vi "Dashboard Main.vi"() -> ()   [LabVIEW 2015]
uses:
  Common Code/Auton Command Cluster.ctl
  Common Code/Auton File Lists.ctl
  Vision/Camera Types.ctl
  Common Code/Goal Vision Packet.ctl
  <vilib>/Rock Robotics/WPI/Camera/WPI_CameraSettings Read MJPG.ctl
  <vilib>/Rock Robotics/WPI/Camera/WPI_CameraImageSize.ctl
  Common Code/Encoder Values Super Cluster.ctl
  Common Code/Encoder Values.ctl
  Common Code/Power and Diagnostic Data.ctl
  Common Code/Utilities/PDP Data.ctl
  Common Code/Utilities/PCM Data.ctl
  Common Code/IMU Data.ctl
  navX.Library.v2/navX Library v2/TypeDefs/Flags/Z900_navX_Flags_CalibrationStatusTypeDef.ctl
  navX.Library.v2/navX Library v2/TypeDefs/Flags/Z900_navX_Flags_OpStatusTypeDef.ctl
  Common Code/Intake Status Cluster.ctl
  Common Code/Intake Mode.ctl
  Common Code/Intake States.ctl
  Common Code/Climb Status Cluster.ctl
  Common Code/Climb Mode.ctl
  Common Code/Climb Presets.ctl
  Common Code/Major Loop Times.ctl
  Common Code/Shooter State Cluster.ctl
  Common Code/Shooter State.ctl
  Common Code/Shoot Modes Enum.ctl
  Common Code/Shot Type.ctl
  Common Code/Drivetrain Settings.ctl
  Common Code/Shooter Presets.ctl
  Common Code/Shot Presets.ctl
  Common Code/Intake Presets.ctl
  Common Code/Drivetrain Output Range.ctl
  Common Code/Ultrasonic Data.ctl
  Common Code/Autonomous Presets.ctl
  Common Code/Robot Name.ctl
  Common Code/Encoder Control.ctl
  Common Code/Drivetrain Status Cluster.ctl
  Common Code/Drivetrain Modes.ctl
  Common Code/Dist Drive Status.ctl
  Common Code/Auto Shift Cluster.ctl
  Common Code/Dashboard Communication/Dashboard Control Data.ctl
  Common Code/Dashboard Drivetrain Command.ctl
  Common Code/Drivetrain Vision.ctl
  Common Code/Ball Tracking Command Cluster.ctl
  Common Code/Ball Vision Packet.ctl
  Common Code/Tracking Mode.ctl
  Common Code/IntakeEcoderControl.ctl
  Common Code/Enabled Systems.ctl
  Common Code/Dashboard Communication/Dashboard Display Data.ctl
  <vilib>/Rock Robotics/WPI/Dashboard/WPI_DashboardLogging Global.vi
  <vilib>/Utility/inputDevices.llb/keyboardAcquire.vi
  navX.Library.v2/navX Library v2/navX Library v2.lvlib
panel:
  in  "Robot":T1
  in  "Logging Filename":path=path ""
  in  "stop":bool
  out "DumbDashMessage":string="137 values loaded OK"
  in  "Save":bool
  in  "Load":bool
  in  "TCP":refnum<k5>
  in  "Rec Mode":enum32{"Stop", "Record", "Playback"}(radio)
  out "Image Message":string="Timeout in Camera Communications"
  in  "Dashboard Tab":T2(tab)
  out "Auto Shift Enabled?":bool
  out "Gear":dbl
  out "Pressure":dbl
  out "Goal Active? 2":bool
  out "Drivetrain Mode":bool
  out "Intake State":bool
  out "Right RPM":dbl(knob) scale=0.0..5000.0
  out "Left RPM":dbl(knob) scale=0.0..5000.0
  out "Mode":T3(ring)=enum."Disconnected"
  out "Shooter Mode":bool
  out "Gyro":dbl(knob) scale=0.0..360.0 scale format="%#.7g"
  out "Climb Mode":bool
  out "Intake Mode":bool
  out "Shooter State":bool
  out "Camera IP":string="0.0.0.0"
  out "Robot IP":string="0.0.0.0"
  out "Angle Ready?":bool
  out "RPM Ready?":bool
  out "Vision Ready?":bool
  out "Ball Loaded?":bool
  out "Shooter Ready?":bool
  out "Front Camera Display":T4(plugin-control)
  in  "Camera Mode":u16(ring)=3 items=["Camera Off", "USB Camera SW", "USB Camera HW", "IP Camera"]
  out "FPS":dbl
  out "Bandwidth (Mbps)":dbl
  out "navX Calibration Status":T5 items=["IMU_CAL_STATE_MASK"=3, "IMU_CAL_STATE_INPROGRESS"=0, "IMU_CAL_STATE_ACCUMULATE"=1, "IMU_CAL_STATE_COMPLETE"=2]
  out "Front Camera Display 2":T4(plugin-control)
  out "Line Number":i32
  in  "Auton Presets":T6
  out "Auton Command Cluster":T7
  out "Auton File Lists":T8
  in  "Auto-Shift":T9
  in  "Encoder Settings":T10
  in  "Drivetrain Settings":T11={"Gyro Tolerance"=6.0, "Throttle Ramp (ms)"=250.0, "Kv"=0.0, "Ka"=0.0, "Feed Forward P"=1.0, "Feed Forward D"=0.0, "Goal Vision PID gains"={"proportional gain (Kc)"=0.8, "integral time (Ti, min)"=0.05, "derivative time (Td, min)"=0.003}, "Goal Detection Window"=12.0, "Creep Rate"=0.0, "Vision Throttle Threshold"=0.0, "Min Turn Output"=0.0, "Left Batter Angle"=0.0, "Right Batter Angle"=0.0} {"Goal Vision PID gains"."derivative time (Td, min)" format="%.5f"; "Goal Vision PID gains"."integral time (Ti, min)" format="%.3f"; "Goal Vision PID gains"."proportional gain (Kc)" format="%.3f"}
  in  "Goal Output Range":cluster{"output high":dbl, "output low":dbl}={"output high"=0.8, "output low"=-0.8}
  out "Encoder Values":T12
  in  "Steer PID output":cluster{"output high":dbl, "output low":dbl}
  in  "Steer PID gains":T14
  out "Drivetrain Status Cluster":T15={"Modes"=enum."Manual", "Y (Throttle)"=0.0, "X (Steer)"=0.0, "Gyro In Range?"=FALSE, "Distance Drive Finished?"=FALSE, "Stop Eject Lockout"=FALSE, "Dist Drive Status"={"Y In Range"=FALSE, "X In Range"=FALSE, "Gyro In Range"=FALSE, "Y Dist"=0.0, "X Dist"=0.0, "Gyro"=0.0}, "Y Target"=0.0, "Heading Target"=0.0, "Vision Target Aligned?"=FALSE, "Gear"=0.0, "1st Gear Time"=0.0, "2nd Gear Time"=0.0, "1st Gear Shifts"=0.0, "2nd Gear Shifts"=0.0} {"2nd Gear Time" scale=0.0..135.0; "1st Gear Time" scale=0.0..135.0}
  in  "Shooter Presets":T18={"Batter Shot"={"L"=1450.0, "R"=1450.0, "A"=69.0}, "Deep Middle"={"L"=0.0, "R"=0.0, "A"=0.0}, "Manual Shot"={"L"=1000.0, "R"=1000.0, "A"=0.0}, "Left Ticks Per Rotation"=-409.6, "Right Ticks Per Rotation"=409.6, "Low Bar Shot"={"L"=2100.0, "R"=2100.0, "A"=42.0}, "Shooter RPM Tolerance"=100.0, "Trigger Power"=0.9, "Fire from Load Delay"=250, "Max Angle"=80.0, "Min Angle"=42.0, "Angle PID gains"={"P"=1.0, "I"=0.0, "D"=0.002}, "Angle Output"={"output high"=0.5, "output low"=-0.5}, "Shooter Angle Tolerance"=3.0, "Vision Shoot x^2"=0.0, "Vision Shoot x"=0.0, "Feed Forward Max Accel"=160.57, "Feed Forward Kv"=0.000217, "Backwards Trigger"=-0.6, "Shot Finish Delay (ms)"=250.0, "Angle Max Current"=40.0, "Angle Current Trip Time"=500.0, "Intake Angle"=80.0, "Vision Shoot c"=0.0, "Reset?"=FALSE, "Button Release Delay"=0.0, "Angle Pot x"=7.0746, "Angle Pot c"=33.439, "Ignore Angle?"=FALSE, "Max RPM"=4600.0, "Safty Frist Angle"=44.0, "Intake Danger Height"=35.0, "Angle Pot B"=0, "Angle Pot M"=12.0, "FF Finish RPM"=0.0, "RPM PID Right"={"P"=0.17, "I"=0.0, "D"=0.0, "FF"=0.036}, "RPM PID Left"={"P"=0.18, "I"=0.0, "D"=0.0, "FF"=0.037}, "Backwards RPM"=-300.0, "Vision RPM"=0.0, "Run Wheels Backward Delay"=0, "Cleat Shot"={"L"=0.0, "R"=0.0, "A"=0.0}, "Vision Far RPM"=0.0, "Vision Far Distance"=0.0, "Vision Far Angle"=0.0}
  out "Shooter State Cluster":T20 {"Trigger Output" scale=-1.0..1.0; "Angle Motor Output" scale=-1.0..1.0; "Right RPM" scale=0.0..5000.0; "Left RPM" scale=0.0..5000.0}
  in  "Intake Presets":T24={"Intake Speed"=0.8, "Outake Speed"=-0.8, "Low Height"=5.0, "Half Height"=55.0, "High Idle Height"=90.0, "Angle Speed"=0.0, "Angle Tolerance"=5.0, "Encoder Scale"=0.001478, "Load Height"=4.0, "Output Range"={"output high"=0.4, "output low"=-0.4}, "Rotation Power Max/Min"=0.5, "MaxCurrent"=40.0, "Intake Trip Time"=500.0, "Idle Height"=27.0, "Max Height"=90.0, "Reset Encoders?"=FALSE, "PID gains"={"proportional gain (Kc)"=1.0, "integral time (Ti, min)"=0.0, "derivative time (Td, min)"=0.003}, "Intake Stop Delay"=0, "Settle Time"=0.0, "Settle Wait Time"=0.0, "Pull Up Delay"=0.0} {"Pull Up Delay" format="%#_7g"; "Settle Wait Time" format="%#_7g"; "Settle Time" format="%#_7g"; "Intake Stop Delay" format="%#_7g"; "Max Height" format="%#_7g"; "Idle Height" format="%#_7g"; "Intake Trip Time" format="%#_7g"; "MaxCurrent" format="%#_7g"; "Rotation Power Max/Min" format="%#_7g"; "Load Height" format="%#_7g"; "Encoder Scale" format="%#_7g"; "Angle Tolerance" format="%#_7g"; "Angle Speed" format="%#_7g"; "High Idle Height" format="%#_7g"; "Half Height" format="%#_7g"; "Low Height" format="%#_7g"; "Outake Speed" format="%#_7g"; "Intake Speed" format="%#_7g"}
  out "Intake Status Cluster":T26
  in  "Climb Presets":T29={"Pull Power"=0.0, "Extend Power"=1.0}
  out "Climb Status Cluster":T30
  in  "Pressure B":dbl
  in  "Pressure M":dbl=22.0
  out "Pressure Sensor Voltage":dbl
  out "IMU Data":T32 {"OP Status" items=["INITIALIZING", "SELFTEST_IN_PROGRESS", "ERROR", "IMU_AUTOCAL_IN_PROGRESS", "NORMAL"]; "Calibration Status" items=["IMU_CAL_STATE_MASK"=3, "IMU_CAL_STATE_INPROGRESS"=0, "IMU_CAL_STATE_ACCUMULATE"=1, "IMU_CAL_STATE_COMPLETE"=2]}
  out "Gyro 2":dbl(knob) scale=0.0..360.0 scale format="%#.7g"
  out "Ultrasonic Data":T34
  out "Ball Cam Active?":bool
  out "Camera Display 2":T4(plugin-control)
  in  "Aspect Fudge Factor":dbl=1.0
  in  "Score Threshold 2":dbl=75.0 format="%#_13g"
  out "Goal Display":T4(plugin-control)
  out "Found Targets":T35(array[cluster]) {"Normalized Rect"."Numeric 5" format="%#_2g"; "Normalized Rect"."Numeric 3" format="%#_2g"; "Normalized Rect"."Numeric 2" format="%#_2g"; "Normalized Rect"."Numeric" format="%#_2g"}
  in  "Camera Type":T36=enum."1013"
  out "Goal Vision Packet":T37
  in  "Goal Camera Settings":T38={"fps"=30, "compression"=30, "Image Size"=enum."320x240"}
  in  "File number":i32
  in  "Use Goal File?":bool
  in  "Color Components":T40={"Hue"={34.0, 185.0}, "Sat"={0.0, 181.0}, "Val"={142.0, 255.0}} {"Val" scale=0.0..255.0; "Sat" scale=0.0..255.0; "Hue" scale=0.0..255.0 scale format="%#_3g"}
  out "Goal Active?":bool
  in  "Camera Mode 2":u16(ring) items=["Camera Off", "USB Camera SW", "USB Camera HW", "IP Camera"]
  out "FPS 2":dbl
  out "Bandwidth (Mbps) 2":dbl
  in  "Ball Camera Settings":T38={"fps"=30, "compression"=30, "Image Size"=enum."320x240"}
  out "Front Camera Display 3":T4(plugin-control)
  in  "Vision Timeout":dbl
  out "Power and Diagnostic Data":T41
  out "Control Info":T44
  out "Status Info":T45
  out "DS TCP":T46={"Error Strings"="", "Disable Counts"={0, 0}, "Rail Faults"={0, 0, 0}, "Robot IP"="0.0.0.0", "DB Mode"=4, "Event Info"={"Name"="", "Type"=0, "Number"=0, "Replay"=0}, "Camera Addr"="0.0.0.0"}
  out "Robot Metrics":T47
  out "Loop Times":T48
  # "USB Cam"
  # "Axis Cam"
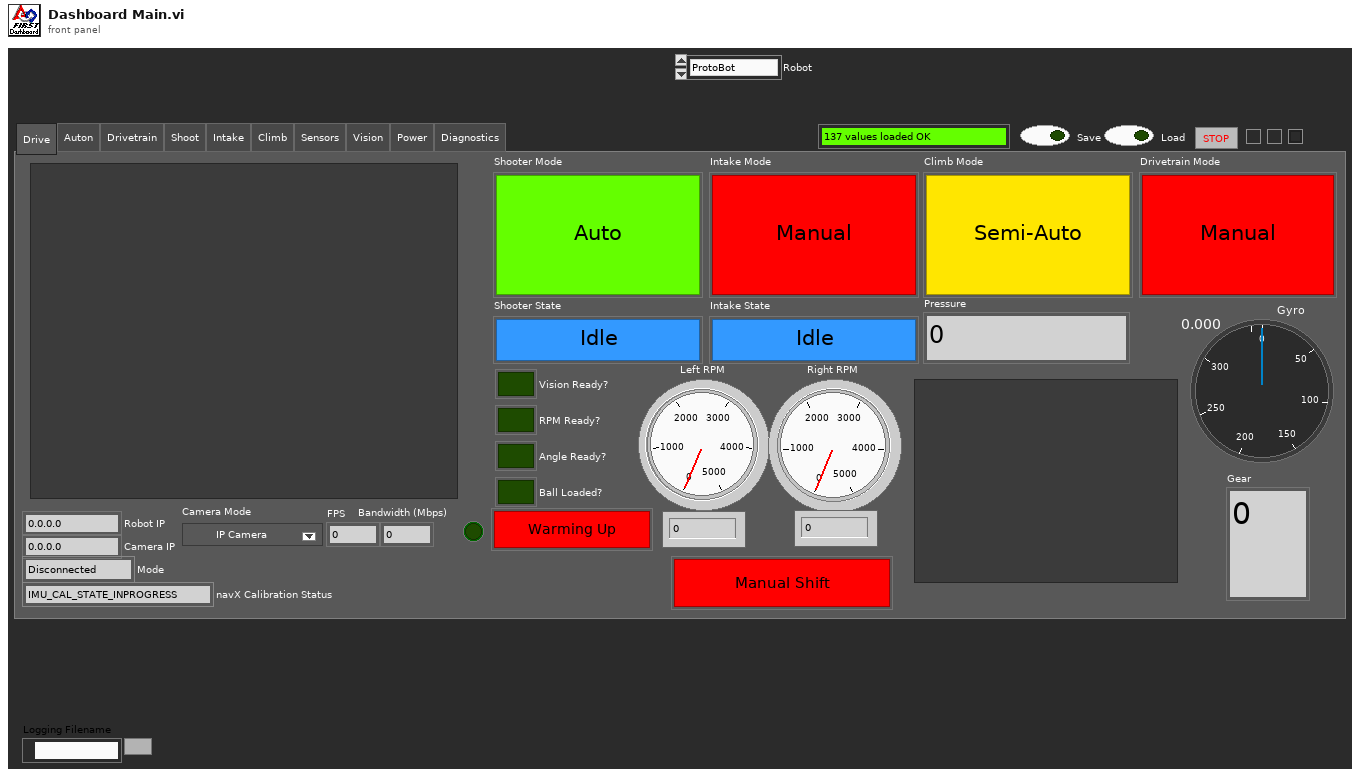
[diagram p1: front panel]
types:
  T1 = typedef "Robot Name.ctl" = enum16{"ProtoBot", "Main Robot", "Practice Robot"}
  T2 = enum32{"Drive", "Auton", "Drivetrain", "Shoot", "Intake", "Climb", "Sensors", "Vision", "Power", "Diagnostics"}
  T3 = enum8{"Tele-Op Disabled", "Tele-Op Enabled", "Auto Disabled", "Auto Enabled", "Test Disabled", "Test Enabled", "Disconnected", "No Code", "E-Stop"}
  T4 = typedef "IMAQ Image.ctl" = refnum<image>
  T5 = typedef "navX Library v2.lvlib/Z900_navX_Flags_CalibrationStatusTypeDef.ctl" = u8
  T6 = typedef "Autonomous Presets.ctl" = cluster{"Pitch Limit":dbl, "Roll Limit":dbl, "Start Position":dbl, "Cross Position":dbl}
  T7 = typedef "Auton Command Cluster.ctl" = cluster{"Command ID":i32, "maxTime":dbl, "Y Distance":dbl, "Heading":dbl, "Throttle":dbl, "Async":dbl, "Velocity":dbl, "Acceleration":dbl, "To":dbl, "Condition":dbl, "Shot Type":dbl, "Left RPM":dbl, "Override RPM":i32, "Override Angle":i32, "Right RPM":dbl, "Angle":dbl, "Intake Mode":i32, "Intake Cmd":i32, "Intake O":i32, "Eject O":i32, "Angle O":i32, "Arm O":i32, "Intake Speed":dbl, "Eject Speed":dbl, "Arm Angle":dbl, "Arm Speed":dbl, "Intake?":i32, "Eject?":i32, "Left":dbl, "Right":dbl, "Pivot Speed":dbl, "Y Dist":dbl, "Position":dbl, "Desired Position":i32, "Shooter Mode":dbl, "Shooter Command":dbl}
  T8 = typedef "Auton File Lists.ctl" = cluster{"Current Queue":string, "General Scripts":string, "Defense Scripts":string, "Movement Scripts":string}
  T9 = typedef "Auto Shift Cluster.ctl" = cluster{"Delay":dbl, "Speed Thresh":dbl, "Upshift Accel":dbl, "Upshift Throttle":dbl, "Upshift Throttle Accel":dbl, "Downshift Throttle":dbl, "Downshift Throttle Accel":dbl}
  T10 = typedef "Encoder Control.ctl" = cluster{"Right Tick Constant":dbl, "Left Tick Constant":dbl, "Reset?":bool, "Y Dist":cluster{"PID gains":cluster{"proportional gain (Kc)":dbl, "integral time (Ti, min)":dbl, "derivative time (Td, min)":dbl}}, "Y Stop Thresh":dbl, "Y Stop Speed":dbl}
  T11 = typedef "Drivetrain Settings.ctl" = cluster{"Gyro Tolerance":dbl, "Throttle Ramp (ms)":dbl, "Kv":dbl, "Ka":dbl, "Feed Forward P":dbl, "Feed Forward D":dbl, "Goal Vision PID gains":cluster{"proportional gain (Kc)":dbl, "integral time (Ti, min)":dbl, "derivative time (Td, min)":dbl}, "Goal Detection Window":dbl, "Creep Rate":dbl, "Vision Throttle Threshold":dbl, "Min Turn Output":dbl, "Left Batter Angle":dbl, "Right Batter Angle":dbl}
  T12 = typedef "Encoder Values Super Cluster.ctl" = cluster{"Left Encoder":T13, "Right Encoder":T13}
  T13 = typedef "Encoder Values.ctl" = cluster{"Distance":dbl, "Speed":dbl, "Ticks":dbl}
  T14 = cluster{"proportional gain (Kc)":dbl, "integral time (Ti, min)":dbl, "derivative time (Td, min)":dbl}
  T15 = typedef "Drivetrain Status Cluster.ctl" = cluster{"Modes":T16, "Y (Throttle)":dbl, "X (Steer)":dbl, "Gyro In Range?":bool, "Distance Drive Finished?":bool, "Stop Eject Lockout":bool, "Dist Drive Status":T17, "Y Target":dbl, "Heading Target":dbl, "Vision Target Aligned?":bool, "Gear":dbl, "1st Gear Time":dbl, "2nd Gear Time":dbl, "1st Gear Shifts":dbl, "2nd Gear Shifts":dbl}
  T16 = typedef "Drivetrain Modes.ctl" = enum16{"Tank", "Climb", "Manual", "Goal Vision Targeting", "PID Distance Drive", "Hybrid", "Gyro Steer"}
  T17 = typedef "Dist Drive Status.ctl" = cluster{"Y In Range":bool, "X In Range":bool, "Gyro In Range":bool, "Y Dist":dbl, "X Dist":dbl, "Gyro":dbl}
  T18 = typedef "Shooter Presets.ctl" = cluster{"Batter Shot":T19, "Deep Middle":T19, "Manual Shot":T19, "Left Ticks Per Rotation":dbl, "Right Ticks Per Rotation":dbl, "Low Bar Shot":T19, "Shooter RPM Tolerance":dbl, "Trigger Power":dbl, "Fire from Load Delay":i32, "Max Angle":dbl, "Min Angle":dbl, "Angle PID gains":cluster{"P":dbl, "I":dbl, "D":dbl}, "Angle Output":cluster{"output high":dbl, "output low":dbl}, "Shooter Angle Tolerance":dbl, "Vision Shoot x^2":dbl, "Vision Shoot x":dbl, "Feed Forward Max Accel":dbl, "Feed Forward Kv":dbl, "Backwards Trigger":dbl, "Shot Finish Delay (ms)":dbl, "Angle Max Current":dbl, "Angle Current Trip Time":dbl, "Intake Angle":dbl, "Vision Shoot c":dbl, "Reset?":bool, "Button Release Delay":dbl, "Angle Pot x":dbl, "Angle Pot c":dbl, "Ignore Angle?":bool, "Max RPM":dbl, "Safty Frist Angle":dbl, "Intake Danger Height":dbl, "Angle Pot B":i32, "Angle Pot M":dbl, "FF Finish RPM":dbl, "RPM PID Right":cluster{"P":dbl, "I":dbl, "D":dbl, "FF":dbl}, "RPM PID Left":cluster{"P":dbl, "I":dbl, "D":dbl, "FF":dbl}, "Backwards RPM":dbl, "Vision RPM":dbl, "Run Wheels Backward Delay":u32, "Cleat Shot":T19, "Vision Far RPM":dbl, "Vision Far Distance":dbl, "Vision Far Angle":dbl}
  T19 = typedef "Shot Presets.ctl" = cluster{"L":dbl, "R":dbl, "A":dbl}
  T20 = typedef "Shooter State Cluster.ctl" = cluster{"State":T21, "Left RPM":dbl, "Right RPM":dbl, "Shooter Ready?":bool, "Ball Loaded?":bool, "Current Angle":dbl, "Angle Motor Output":dbl, "Trigger Output":dbl, "Angle Ready?":bool, "RPM Ready?":bool, "Vision Ready?":bool, "Ball Loaded?":bool, "Mode":T22, "Shot Type":T23, "Pot Height":dbl, "Current Tripped Forward?":bool, "Current Tripped Backward?":bool, "Right Servo":i32, "Left Servo":i32, "IR Override":bool, "Intake Danger?":bool, "Intake Angle Ready?":bool}
  T21 = typedef "Shooter State.ctl" = enum16{"Idle", "Settle Ball", "Warmup", "Shooter Ready", "Shoot"}
  T22 = typedef "Shoot Modes Enum.ctl" = enum16{"Manual", "Safe", "Auto"}
  T23 = typedef "Shot Type.ctl" = enum16{"Batter Shot", "Corner Shot", "Cleat Shot", "Vision Shot", "Deep Middle Shot"}
  T24 = typedef "Intake Presets.ctl" = cluster{"Intake Speed":dbl, "Outake Speed":dbl, "Low Height":dbl, "Half Height":dbl, "High Idle Height":dbl, "Angle Speed":dbl, "Angle Tolerance":dbl, "Encoder Scale":dbl, "Load Height":dbl, "Output Range":T25, "Rotation Power Max/Min":dbl, "MaxCurrent":dbl, "Intake Trip Time":dbl, "Idle Height":dbl, "Max Height":dbl, "Reset Encoders?":bool, "PID gains":cluster{"proportional gain (Kc)":dbl, "integral time (Ti, min)":dbl, "derivative time (Td, min)":dbl}, "Intake Stop Delay":u32, "Settle Time":dbl, "Settle Wait Time":dbl, "Pull Up Delay":dbl}
  T25 = typedef "Drivetrain Output Range.ctl" = cluster{"output high":dbl, "output low":dbl}
  T26 = typedef "Intake Status Cluster.ctl" = cluster{"Roller Power":dbl, "Angle Power":dbl, "Intake Mode":T27, "Intake States":T28, "Rollers Active?":bool, "Current Height":dbl, "Target Height":dbl, "Encoder Raw Position":dbl, "Forward Tripped?":bool, "Backward Tripped?":bool, "Override IR?":bool}
  T27 = typedef "Intake Mode.ctl" = enum16{"Safe", "Auto", "Manual"}
  T28 = typedef "Intake States.ctl" = enum16{"Idle", "Set roller speed", "Move to angle", "Go Hard or Go Home", "Ball Settle"}
  T29 = typedef "Climb Presets.ctl" = cluster{"Pull Power":dbl, "Extend Power":dbl}
  T30 = typedef "Climb Status Cluster.ctl" = cluster{"Pull Power":dbl, "Unpin Power":dbl, "PTO Engaged?":bool, "Climb Mode":T31}
  T31 = typedef "Climb Mode.ctl" = enum16{"Auto", "Semi-Auto", "Manual"}
  T32 = typedef "IMU Data.ctl" = cluster{"Pitch":sgl, "Roll":sgl, "Yaw":sgl, "Data Valid?":bool, "Temp":sgl, "MOVING":bool, "YAW_STABLE":bool, "Accel X":sgl, "Accel Y":sgl, "Accel Z":sgl, "Accel Magnitude":sgl, "Pitch Rate":sgl, "Roll Rate":sgl, "Yaw Rate":sgl, "NavX Opened?":bool, "Calibration Status":T5, "OP Status":T33}
  T33 = typedef "navX Library v2.lvlib/Z900_navX_Flags_OpStatusTypeDef.ctl" = u8
  T34 = typedef "Ultrasonic Data.ctl" = cluster{"Left Ultrasonic":dbl, "Right Ultrasonic":dbl}
  T35 = cluster{"Distance (ft)":dbl, "Center":cluster{dbl, dbl}, "Normalized Rect":cluster{"Numeric":dbl, "Numeric 2":dbl, "Numeric 3":dbl, "Numeric 5":dbl}}[]
  T36 = typedef "Camera Types.ctl" = enum16{"206", "1011", "1013", "MS HD3000 square", "MS HD3000 640x480"}
  T37 = typedef "Goal Vision Packet.ctl" = cluster{"Distance":dbl, "Center X":dbl, "Center Y":dbl, "Found Target?":bool, "Robot Center":dbl, "Angle":dbl}
  T38 = typedef "WPI_CameraSettings Read MJPG.ctl" = cluster{"fps":i32, "compression":i32, "Image Size":T39}
  T39 = typedef "WPI_CameraImageSize.ctl" = enum16{"640x480", "320x240", "160x120", "Custom"}
  T40 = cluster{"Hue":cluster{dbl, dbl}, "Sat":cluster{dbl, dbl}, "Val":cluster{dbl, dbl}}
  T41 = typedef "Power and Diagnostic Data.ctl" = cluster{"PDP Data":T42, "PCM Data":T43, "roboRIO input voltage (V)":dbl, "roboRIO input current (A)":dbl, "3.3V Rail Short":bool, "5 V Rail Short":bool, "6 V Rail Short":bool, "roboRIO Brownout":bool, "Outputs Enabled?":bool}
  T42 = typedef "PDP Data.ctl" = cluster{"Battery Voltage":sgl, "Temperature (degrees C)":sgl, "Internal Battery R (Ohms)":sgl, "Energy (J)":sgl, "Power (W)":sgl, "Total Current (A)":sgl, "Battery Voltage Fault":bool, "Temperature Fault":bool, "Hardware Fault":bool, "Currents":cluster{"[0]":sgl, "[1]":sgl, "[2]":sgl, "[3]":sgl, "[4]":sgl, "[5]":sgl, "[6]":sgl, "[7]":sgl, "[8]":sgl, "[9]":sgl, "[10]":sgl, "[11]":sgl, "[12]":sgl, "[13]":sgl, "[14]":sgl, "[15]":sgl}, "Current Faults":cluster{"[0]":bool, "[1]":bool, "[2]":bool, "[3]":bool, "[4]":bool, "[5]":bool, "[6]":bool, "[7]":bool, "[8]":bool, "[9]":bool, "[10]":bool, "[11]":bool, "[12]":bool, "[13]":bool, "[14]":bool, "[15]":bool}}
  T43 = typedef "PCM Data.ctl" = cluster{"Compressor Fault":bool, "Solenoid Fault":bool, "Compressor Enabled":bool, "Hardware Fault":bool, "Compressor Current":dbl}
  T44 = cluster{"Control Bits":cluster{"TestMode":bool, "Autonomous":bool, "Enabled":bool, "FMS Present":bool, bool, bool, bool, "E-Stop":bool}, "Team Station ":u8, "Countdown":sgl, "Joystick Values":cluster{"Axes":dbl[], "Buttons":bool[], "POVs":i16[]}[]}
  T45 = cluster{"Status bits":cluster{"Test Mode":bool, "Autonomous":bool, "Enabled":bool, "Code Start":bool, "Brownout":bool, "Reserved 2":bool, "Reserved 3":bool, "E-Stop":bool}, "Code Trace":cluster{"Disabled":bool, "TeleOp":bool, "Auto":bool, "Test":bool}, "Controller Type":enum16{"unknown", "cRIO", "roboRio"}, "Code?":enum16{"unknown", "noCode", "code"}, "Battery V":dbl}
  T46 = cluster{"Error Strings":string, "Disable Counts":cluster{u16, u16}, "Rail Faults":cluster{u16, u16, u16}, "Robot IP":string, "DB Mode":u8, "Event Info":cluster{"Name":string, "Type":u8, "Number":u16, "Replay":u8}, "Camera Addr":string}
  T47 = cluster{"Storage":cluster{"Disk Free":u64, "RAM Block":u32, "RAM free":u32}, "CPU Utilization":cluster{"CPU % ISR":sgl, "CPU % Time Crit":sgl, "CPU % Timed Str":sgl, "CPU % High":sgl, "CPU % Above":sgl, "CPU % Normal":sgl, "CPU % Low":sgl}, "CAN":cluster{"% Bus Utilization":sgl, "Bus Off Cnt":u32, "TX_FIFO Full Cnt":u32, "Receive Error Cnt":u8, "Transmit Error Cnt":u8}, "HID":cluster{"HID Outputs":u32, "Rumble Low":u16, "Rumble High":u16}[]}
  T48 = typedef "Major Loop Times.ctl" = cluster{"DT Loop Timer":u32, "Shooter Loop Timer":u32, "Intake Loop Timer":u32, "US Loop Timer":u32, "Auton File Loop Timer":u32}
  T49 = typedef "Image Type" = u32
  T50 = typedef "NI_LVConfig.lvlib/Config Data RefNum.ctl" = refnum<k1>
  T51 = cluster{cluster{dbl, dbl}, cluster{dbl, dbl}, cluster{dbl, dbl}}
  T52 = cluster{"Bounding box":cluster{"left":dbl, "top":dbl, "right":dbl, "bottom":dbl}, "Aspect Ratio":dbl, "Area to CH":dbl, "X Mask":dbl, "Y Mask":dbl, "Moment":dbl}[]
  T53 = cluster{"Distance (ft)":dbl, "Center":cluster{dbl, dbl}, "Normalized Rect":cluster{"Numeric":dbl, "Numeric 2":dbl, "Numeric 3":dbl, "Numeric 5":dbl}}
  T54 = typedef "Dashboard Display Data.ctl" = cluster{"Auton Command Cluster":T7, "Auton File Lists":T8, "Drivetrain Status Cluster":T15, "Encoder Values":T12, "IMU Data":T32, "Power and Diagnostic Data":T41, "Gyro":dbl, "Shooter State Cluster":T20, "Intake Status Cluster":T26, "Ultrasonic Data":T34, "Climb Status Cluster":T30, "Loop Times":T48, "Pressure":dbl, "Pressure Voltage":dbl, "Auton Line Number":i32, "Autoshift Enabled":bool}
  T55 = typedef "Dashboard Control Data.ctl" = cluster{"Shooter Presets":T18, "Encoder Control":T10, "Steer PID output":cluster{"output high":dbl, "output low":dbl}, " Steer PID gains":cluster{"proportional gain (Kc)":dbl, "integral time (Ti, min)":dbl, "derivative time (Td, min)":dbl}, "Drivetrain Settings":T11, "Vision Packet":T37, "Dashboard Drivetrain Command":T56, "Info/Command Cluster":T58, "Ball Vision Packet":T59, "Intake Presets":T24, "Intake Encoder Control":T61, "Climb Presets":T29, "Goal Output Range":cluster{"output high":dbl, "output low":dbl}, "Enabled Systems":T62, "Auton Presets":T6, "Pressure M":dbl, "Pressure B":dbl, "Vision Timeout":dbl, "Auto-Shift":T9}
  T56 = typedef "Dashboard Drivetrain Command.ctl" = cluster{"Drivetrain Vision":T57}
  T57 = typedef "Drivetrain Vision.ctl" = cluster{"Goal Window":dbl, "Ball Window":dbl}
  T58 = typedef "Ball Tracking Command Cluster.ctl" = cluster{"Distance to Ball":dbl, "Desired Angle":dbl, "Command":enum16{"Turn to Ball", "Turn to Angle", "Get Distance"}, "Pixels from Center":dbl}
  T59 = typedef "Ball Vision Packet.ctl" = cluster{"Ball Detected?":bool, "Distance to Ball":dbl, "Desired Angle":dbl, "Pixels from Center":dbl, "Tracking mode":T60}
  T60 = typedef "Tracking Mode.ctl" = enum16{"Turn to Ball", "Turn to Angle"}
  T61 = typedef "IntakeEcoderControl.ctl" = cluster{"Arm Tick Constant":dbl, "Reset?":bool, "Y Dist":cluster{"PID gains":cluster{"proportional gain (Kc)":dbl, "integral time (Ti, min)":dbl, "derivative time (Td, min)":dbl}}, "Y Stop Thresh":dbl, "Y Stop Speed":dbl}
  T62 = typedef "Enabled Systems.ctl" = cluster{"Shoot":bool, "Intake":bool, "DT":bool, "Gyro":bool, "100ms":bool, "US":bool}
  T63 = cluster{"Image Size":bool, "Image Type":bool, "Pixel Value":bool, "ROI Information":bool, "Zoom Factor":bool}
  T64 = enum16{"0", "1", "2", "3", "4", "5", "6", "7", "8", "9", "A", "B", "C", "D", "E", "F", "G", "H", "I", "J", "K", "L", "M", "N", "O", "P", "Q", "R", "S", "T", "U", "V", "W", "X", "Y", "Z", "F1", "F2", "F3", "F4", "F5", "F6", "F7", "F8", "F9", "F10", "F11", "F12", "F13", "F14", "F15", "ADD", "BACK", "BACKSLASH", "CAPITAL", "COMMA", "DECIMAL", "DELETE", "DIVIDE", "DOWN", "END", "EQUALS", "ESCAPE", "GRAVE (`)", "HOME", "INSERT", "LBRACKET", "LCONTROL", "LEFT", "L ALT", "LSHIFT", "LWIN", "MINUS", "MULTIPLY", "NEXT", "NUMLOCK", "NUMPAD_0", "NUMPAD_1", "NUMPAD_2", "NUMPAD_3", "NUMPAD_4", "NUMPAD_5", "NUMPAD_6", "NUMPAD_7", "NUMPAD_8", "NUMPAD_9", "PAUSE", "PERIOD", "PRIOR (PG UP)", "RBRACKET", "RCONTROL", "RETURN", "RIGHT", "R ALT", "RSHIFT", "RWIN", "SCROLL", "SEMICOLON", "SLASH", "SPACE", "SUBTRACT", "TAB", "UP", "ENTER (num pad)", "' (quote)"}[]
  T65 = typedef "DumbDash Control.ctl" = cluster{"Name":string, "Ref":refnum<vi>, "Type":T66}
  T66 = typedef "DumbDash Control Type.ctl" = enum16{"Invalid", "Number", "Boolean", "String"}
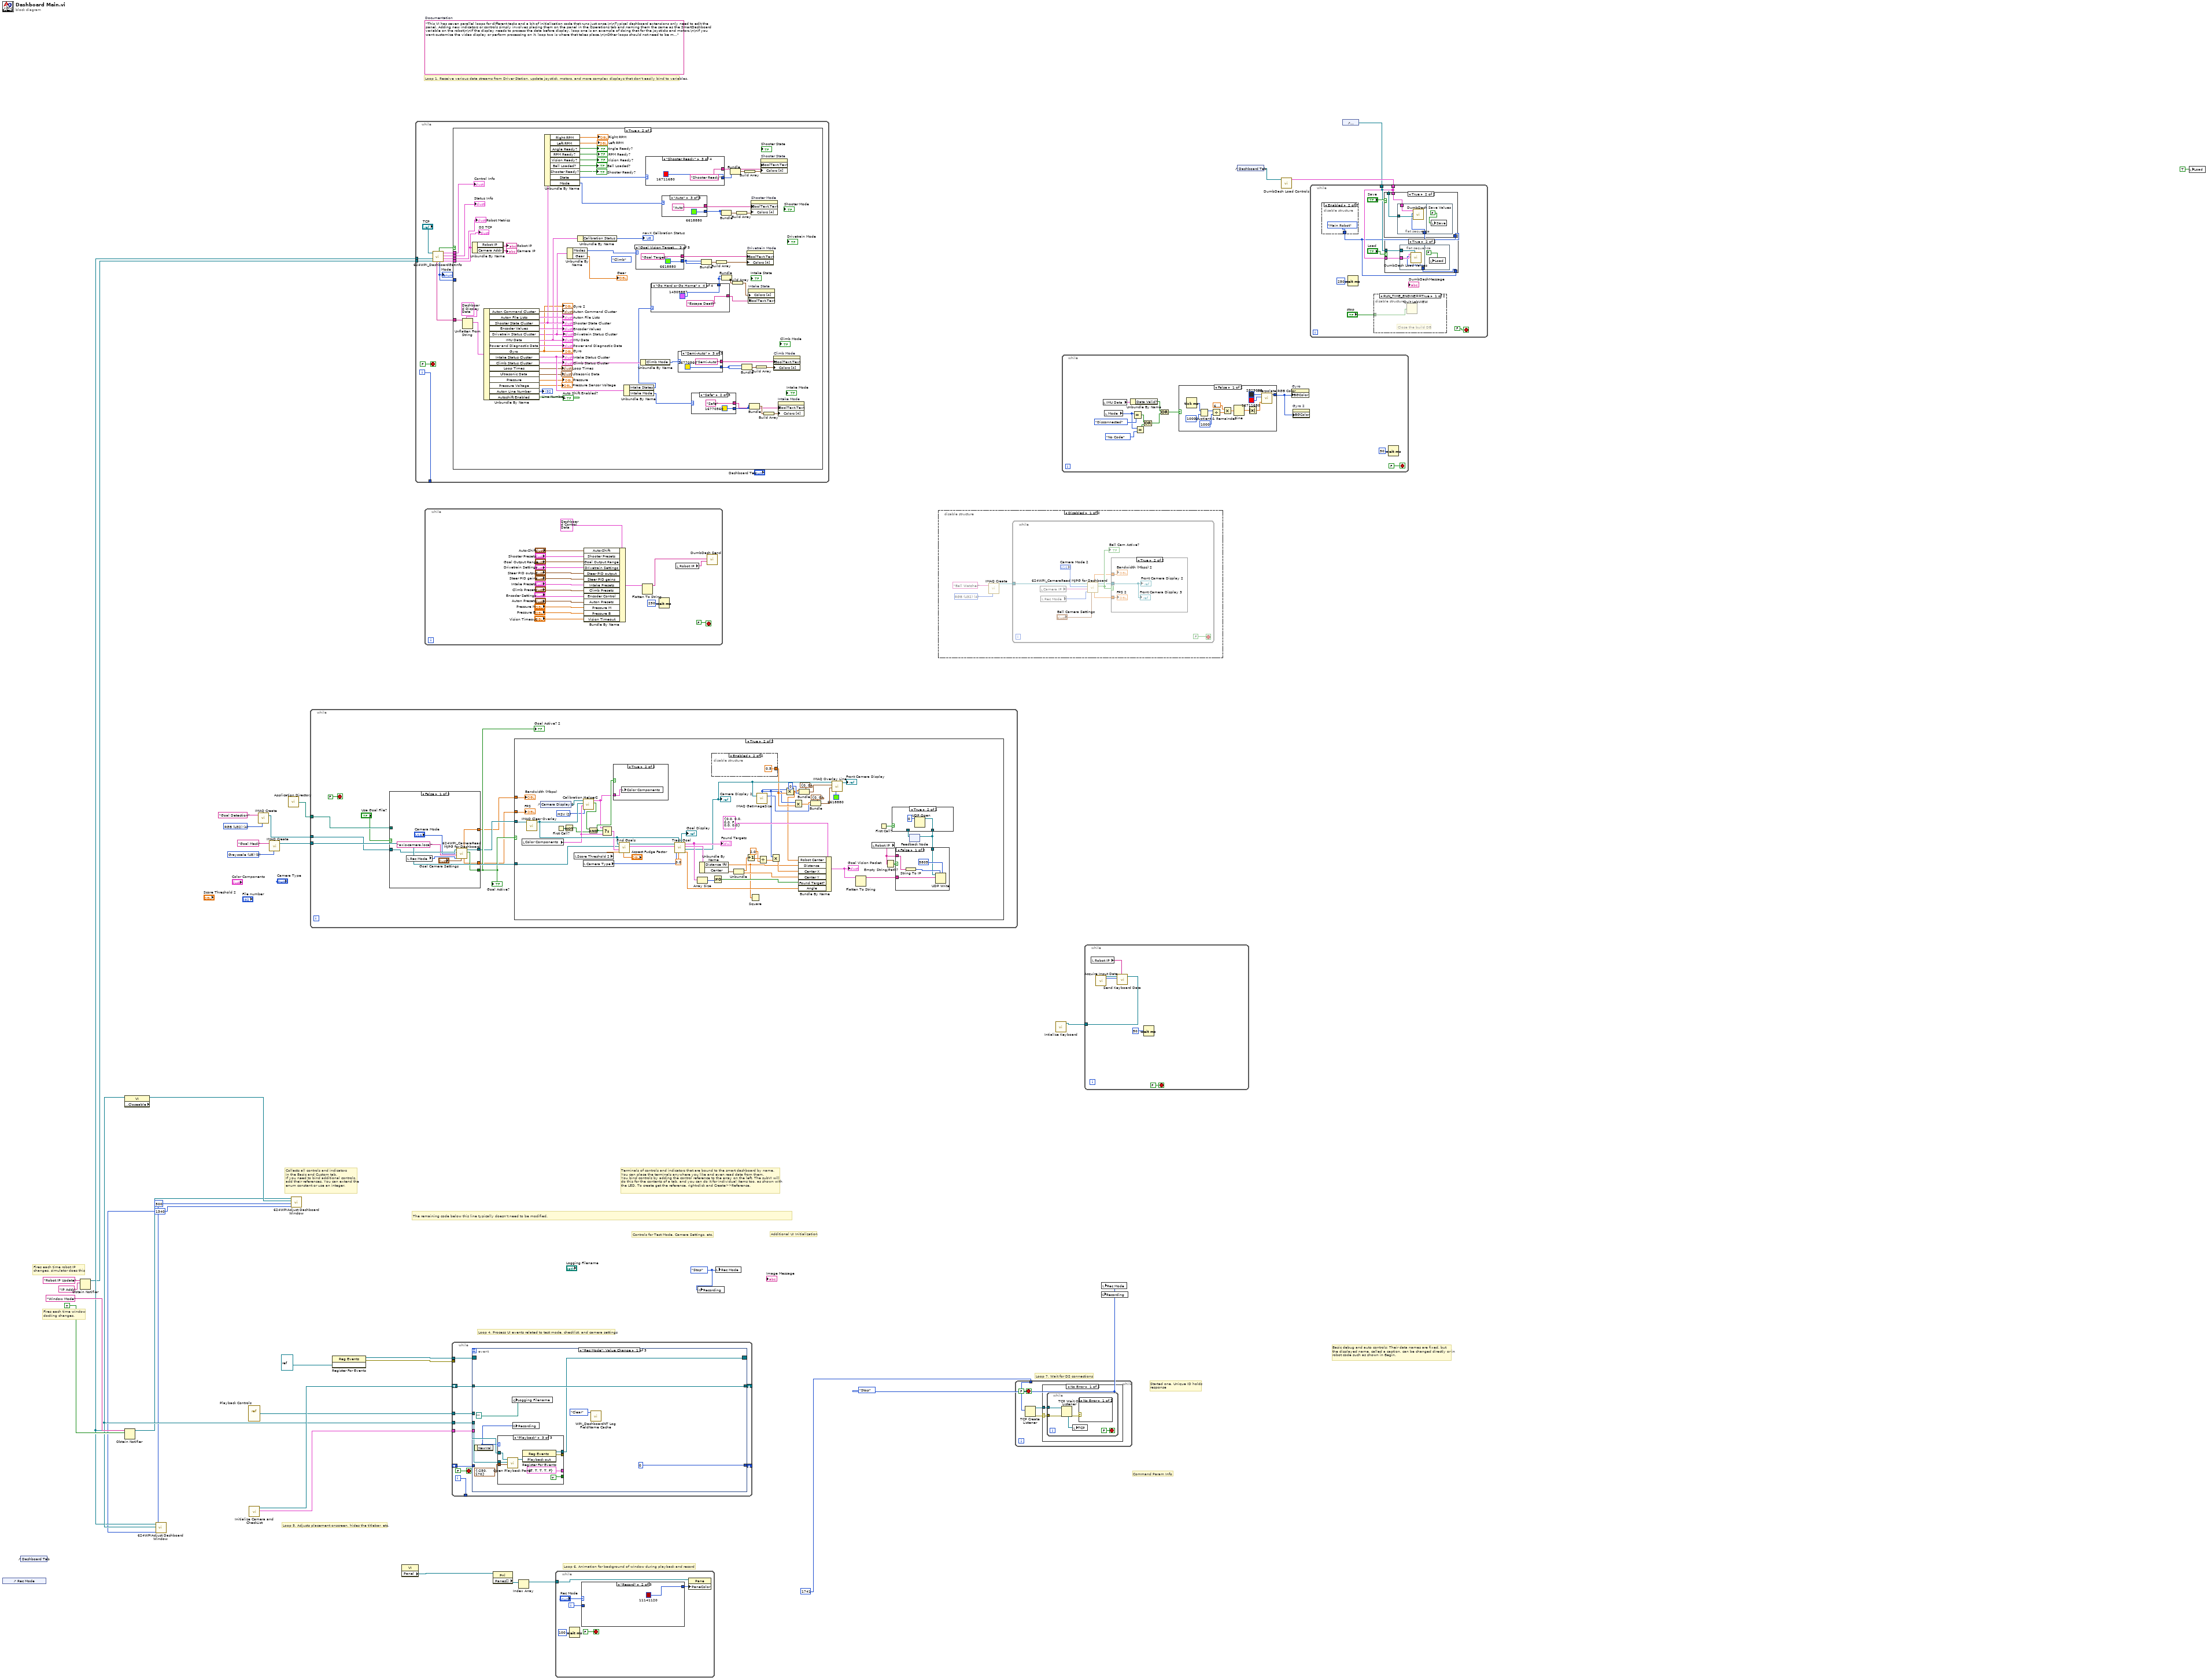
[diagram p0: block diagram]
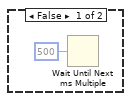
[diagram p2: hidden frame]
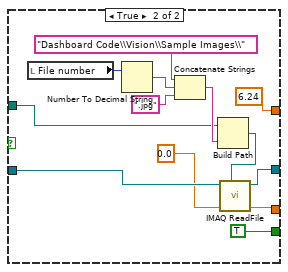
[diagram p4: hidden frame]
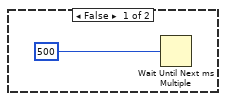
[diagram p5: hidden frame]
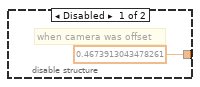
[diagram p9: hidden frame]
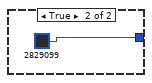
[diagram p10: hidden frame]
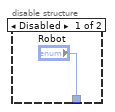
[diagram p11: hidden frame]
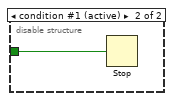
[diagram p12: hidden frame]
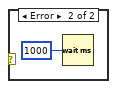
[diagram p15: hidden frame]
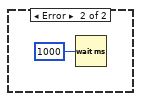
[diagram p16: hidden frame]
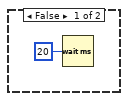
[diagram p17: hidden frame]
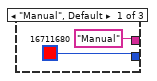
[diagram p18: hidden frame]
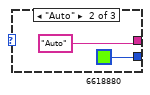
[diagram p19: hidden frame]
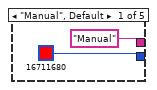
[diagram p20: hidden frame]
diagram:
  w3 = T49 0 items=["Grayscale (U8)", "Grayscale (I16)", "Grayscale (SGL)", "Complex (CSG)", "RGB (U32)", "HSL (U32)", "RGB (U64)", "Grayscale (U16)"] ("Image Type")
  w7 = T49 4 items=["Grayscale (U8)", "Grayscale (I16)", "Grayscale (SGL)", "Complex (CSG)", "RGB (U32)", "HSL (U32)", "RGB (U64)", "Grayscale (U16)"] ("Image Type")
  w10 = enum16{"Stop", "Record", "Playback"}."Stop"
  w15 = 1340
  w16 = 500
  w20 = enum32{"Stop", "Record", "Playback"}."Stop" ("Rec Mode")
  (unwired) "This VI has seven parallel loops for different tasks and a bit of initialization code that runs just once.\n\nTypical dashboard extensions only need to edit the panel. Adding new indicators or controls simply involves placing them on the panel in the Operations tab and naming them the same as the SmartDashboard variable on the robot\n\nIf the display needs to process the data before display, loop one is an example of doing that for the joysticks and motors.\n\nIf you want customize the video display or perform processing on it, loop two is where that takes place.\n\nOther loops should not need to be modified. They are pretty standard, and document the task they perform."  # Documentation
  # "Command Param Info"
  # "Started one, Unique ID holds\nresponse"
  # "Loop 7. Wait for DS connections"
  # "Basic debug and auto controls: Their data names are fixed, but\nthe displayed name, called a caption, can be changed directly or in\nrobot code such as shown in Begin."
  # "Controls for Test Mode, Camera Settings, etc."
  # "Additional UI Initialization"
  # "Loop 6. Animation for background of window during playback and record"
  # "Fires each time robot IP\nchanges, simulator does this"
  # "Fires each time window\ndocking changes."
  # "Collects all controls and indicators\nin the Basic and Custom tab.\nIf you need to bind additional controls,\nadd their references. You can extend the\nenum constant or use an integer."
  # "The remaining code below this line typically doesn't need to be modified."
  # "Loop 4. Process UI events related to test mode, checklist, and camera settings"
  # "Terminals of controls and indicators that are bound to the smart dashboard by name.\nYou can place the terminals anywhere you like and even read data from them.\nYou bind controls by adding the control reference to the array on the left. The subVI will\ndo this for the contents of a tab, and you can do it for individual items too, as shown with\nthe LED. To create get the reference, right-click and Create>>Reference."
  # "Loop 5. Adjusts placement onscreen, hides the titlebar, etc."
  # "Loop 1. Receive various data streams from Driver Station, update joystick, motors, and more complex displays that don't easily bind to variables."
  n1 = control-ref of="Rec Mode"() -> ()  [unwired: 1 out]
  n2 = control-ref of="Dashboard Tab"() -> ()  [unwired: 1 out]
  n3 = Obtain Notifier(name (unnamed)="Robot IP Update", notification data type="IP Addr" ("name (unnamed)")) -> (notifier out=w14:refnum<notifier>)  [unwired: 2 in, 2 out]
  n4 = property class="VI" props=["Front Panel.Closeable"]() -> (reference out=w19:refnum<vi>)  [unwired: 2 in, 2 out]
  n5 = Obtain Notifier(name (unnamed)="Window Mode", notification data type=TRUE) -> (notifier out=w18:refnum<notifier>)  [unwired: 2 in, 2 out]
  n6 = call "624WPIAdjust Dashboard Window.vi"("Width"=w15, "Height"=w16, "VI"=w19, "Notifier in"=w18) -> ()  [unwired: 8 in]
  n7 = vi-ref "Playback Controls.vi"() -> (w24:refnum<vi>)
  n8 = call "Initialize Camera and CheckList.vi"() -> ("Array"=w29:cluster{string[]}[], "File Refnum"=w28:T50)  [unwired: 9 in, 1 out]
  n9 = call "IMAQ Create"("Image Name"="Goal Detection", "Image Type"=w7) -> ("New Image"=w8:T4)  [unwired: 3 in, 1 out]
  n10 = call "IMAQ Create"("Image Name"="Goal Mask", "Image Type"=w3) -> ("New Image"=w5:T4)  [unwired: 3 in, 1 out]
  n11 = call <vilib>:"Application Directory.vi"() -> ("Application Directory"=w2:path)
  n12 = call "624WPIAdjust Dashboard Window.vi"("Width"=w15, "Height"=w16, "VI"=w19, "Notifier in"=w18) -> ()  [unwired: 8 in]
  n13 = while {
    tunnel: w5 -> [w42]
    tunnel: w8 -> [w40]
    tunnel: w2 -> [w38]
    stop <- FALSE stop-if-true
    n14 = case shown="False" "Use Goal File?" {
      tunnel: [w46 TRUE] -> w41
      tunnel: w40 -> [w51 w62]
      tunnel: [w45 w61] -> w39
      tunnel: w38 -> [_ w56]
      tunnel: [w43 6.24 ("Bandwidth (Mbps)")] -> w36
      tunnel: [w44 0.0 ("FPS")] -> w35
      frame False {
        n15 = local read "Rec Mode"() -> (w48:enum32{"Stop", "Record", "Playback"})
        n16 = call "624WPI_CameraRead MJPG for Dashboard.vi"("Camera Settings"="Goal Camera Settings", "Rec Mode"=w48, "Camera IP"="axis-camera.local", "Camera Mode"="Camera Mode", "Refnum in"=w51) -> ("Active"=w46:bool, "Refnum out"=w45:T4, "FPS"=w44:dbl, "Bandwidth (Mbps)"=w43:dbl)  [unwired: 3 in]
      }
      frame True {
        n17 = local read "File number"() -> (w54:i32)
        n18 = Number To Decimal String(number=w54) -> (decimal integer string=w59:string)  [unwired: 1 in]
        n19 = Concatenate Strings("Dashboard Code\\Vision\\Sample Images\\", w59, ".jpg" ("string")) -> (w57:string)
        n20 = Build Path(base path=w56, name or relative path=w57) -> (appended path=w55:path)
        n21 = call "IMAQ ReadFile"("File Path"=w55, "Image"=w62) -> ("Image Out"=w61:T4)  [unwired: 5 in, 4 out]
      }
    }
    "Goal Active?" <- w41
    "Goal Active? 2" <- w41
    n22 = case shown="True" w41 {
      tunnel: w39 -> [_ w118]
      tunnel: w42 -> [_ w99]
      tunnel: w36 -> [_ w107]
      tunnel: w35 -> [_ w106]
      frame False {
        n23 = Wait Until Next ms Multiple(millisecond multiple=u32 500) -> ()  [unwired: 1 out]
      }
      frame True {
        w102 = u16 2 items=["RGB", "HSL", "HSV", "HSI", "CIE L*a*b*", "CIE XYZ"] ("Color Mode")
        n24 = local read "Color Components"() -> (w103:T40)
        n25 = call "IMAQ Clear Overlay"("Image"=w118) -> ("Image Out"=w105:T4)  [unwired: 9 in, 1 out]
        n26 = control-ref of="Camera Display 2"() -> (w104:refnum<vi>)
        n27 = First Call?() -> (First Call?: T/F=w69:bool)
        n28 = Not(x=w69) -> (.not. x?=w68:bool)
        n29 = local read "Score Threshold 2"() -> (w119:dbl)
        n30 = call "Calibration Helper2.vi"("Color Mode"=w102, "Color Components"=w103, "Image"=w105, "Image Ctl Refnum"=w104) -> ("Changed"=w67:bool, "output color"=w65:T51)  [unwired: 6 in]
        n31 = local read "Camera Type"() -> (w115:T36)
        n32 = And(x=w67, y=w68) -> (x .and. y?=w66:bool)
        n33 = Select(t=w65, s=w66, f=w103) -> (s? t:f=w101:T40)
        n34 = case shown="True" w66 {
          tunnel: w65 -> [_ w120]
          frame False {
          }
          frame True {
            n35 = local write "Color Components"(w120) -> ()
          }
        }
        n36 = call "Find Goals.vi"("Aspect Fudge Factor"="Aspect Fudge Factor", "Score Threshold"=w119, "Color"=w101, "Image Dst"=w99, "Image Src"=w105) -> ("Targets"=w117:T52, "Masked Image"=w116:T4)  [unwired: 5 in]
        n37 = call "Track Goal.vi"("Offset"=0.0, "Original Image"=w105, "Camera Type"=w115, "Targets"=w117, "Goal Display"=w116) -> ("Angle Difference"=w81:dbl, "Target Line Masking Out"=w90:T4, "Best Target Available"=w114:T53, "Found Targets"=w109:T35, "Goal Display"=→"Goal Display":T4)  [unwired: 2 in]
        "Found Targets" <- w109
        "Camera Display 2" <- w90
        n38 = Array Size(array=w109) -> (size(s)=w110:i32)
        n39 = Unbundle By Name(w114) -> ("Distance (ft)"=w78:dbl, "Center"=w112:cluster{dbl, dbl})
        n40 = disable-structure shown="Enabled" {
          disable-tunnel: [0.4673913043478261 0.5] -> w89
          frame Disabled {
            # "when camera was offset"
          }
          frame Enabled {
          }
        }
        n41 = Not Equal To 0?(x=w110) -> (x != 0?=w108:bool)
        n42 = Unbundle(w112) -> (w88:dbl, w111:dbl)
        n43 = Increment(x=w88) -> (x+1=w87:dbl)
        n44 = Square(x=w78) -> ()  [unwired: 1 out]
        n45 = call "IMAQ GetImageSize"("Image"=w90) -> ("Y Resolution"=w92:i32, "X Resolution"=w83:i32)  [unwired: 3 in, 1 out]
        n46 = Divide(x=w87, y=2.0) -> (x/y=w85:dbl)
        n47 = Multiply(x=w83, y=w85) -> (x*y=w84:dbl)
        n48 = Multiply(x=w83, y=w89) -> (x*y=w82:dbl)
        n49 = Multiply(x=w83, y=w89) -> (x*y=w95:dbl)
        n50 = Bundle By Name(cluster=T37 {"Distance"=0.0, "Center X"=0.0, "Center Y"=0.0, "Found Target?"=FALSE, "Robot Center"=0.0, "Angle"=0.0}, "Robot Center"=w82, "Distance"=w78, "Center X"=w84, "Center Y"=w111, "Found Target?"=w108, "Angle"=w81) -> (w71:T37)
        "Goal Vision Packet" <- w71
        n51 = Bundle(cluster=cluster{"X":i32, "Y":i32} {"X"=0, "Y"=0} ("Start Point"), "X"=w82, "Y"=0) -> (w94:cluster{"X":i32, "Y":i32})
        n52 = Bundle(cluster=cluster{"X":i32, "Y":i32} {"X"=0, "Y"=0} ("Start Point"), "X"=w95, "Y"=w92) -> (w93:cluster{"X":i32, "Y":i32})
        n53 = call "IMAQ Overlay Line"("Color"=u32 6618880, "End Point"=w93, "Start Point"=w94, "Image"=w90) -> ("Image Out"=→"Front Camera Display":T4)  [unwired: 6 in, 1 out]
        n54 = Flatten To String(anything=w71) -> (data string=w70:string)  [unwired: 3 in, 2 out]
        n55 = local read "Robot IP"() -> (w72:string)
        n56 = First Call?() -> (First Call?: T/F=w75:bool)
        n57 = Empty String/Path?(string/path=w72) -> (empty?=w76:bool)
        n58 = feedback #1() -> (w73:refnum<k16>)  [unwired: 1 in]
        n59 = case shown="True" w75 {
          tunnel: [w121 w123] -> w74
          tunnel: w73 -> [w121 _]
          frame False {
          }
          frame True {
            n60 = UDP Open(11:u16 0 ("port")) -> (port=w123:refnum<k16>)  [unwired: 4 in, 2 out]
          }
        }
        n61 = case shown="False" w76 {
          tunnel: w72 -> [w126 _]
          tunnel: w70 -> [w125 _]
          tunnel: w74 -> [w124 _]
          frame False {
            n62 = String To IP(1:w126) -> (0:w127:u32)
            n63 = UDP Write(address=w127, port or service name=u16 5805, connection ID=w124, data in=w125) -> ()  [unwired: 2 in, 2 out]
          }
          frame True {
            # "The robot IP is not\nready yet, don't try\nto send data"
          }
        }
        n64 = feedback-in #1(w74) -> ()
        "Bandwidth (Mbps)" <- w107
        "FPS" <- w106
      }
    }
  }
  n65 = register-events(refnum<vi> refnum) -> (reference out=w23:refnum<event-registration>, error out=w22:errorcluster)  [unwired: 2 in]
  n66 = property class="VI"() -> ("Panel"=w26:refnum<vi>)  [unwired: 2 in, 2 out]
  n67 = while {
    tunnel: [w141] -> _
    tunnel: w14 -> [w140]
    tunnel: w18 -> [w138]
    i -> [w141]
    stop <- FALSE stop-if-true
    n68 = call "624WPI_DashboardGetInfo.vi"("Binding Refnum"=w140, "Window Mode Notifier"=w138, "TCP Cnx"="TCP") -> ("Power and Errors"=w137:T46, "Robot Metrics"=w136:T47, "Status Info"=w135:T45, "Control Info"=w134:T44, "Robot Mode"=w133:T3, "Process?"=w132:bool, "Custom Dashboard Data"=w131:string)  [unwired: 2 in]
    "Mode" <- w133
    n69 = case shown="True" w132 {
      tunnel: w135 -> [_ w206]
      tunnel: w136 -> [_ w205]
      tunnel: w134 -> [_ w207]
      tunnel: w137 -> [_ w204]
      tunnel: w133 -> [_ _]
      tunnel: w131 -> [_ w201]
      frame False {
        n70 = Wait (ms)(milliseconds to wait=u32 20) -> ()  [unwired: 1 out]
      }
      frame True {
        (unwired) Drivetrain_Modes."Climb" ("Modes")
        n71 = Unflatten From String(type=T54 {"Auton Command Cluster"={"Command ID"=0, "maxTime"=0.0, "Y Distance"=0.0, "Heading"=0.0, "Throttle"=0.0, "Async"=0.0, "Velocity"=0.0, "Acceleration"=0.0, "To"=0.0, "Condition"=0.0, "Shot Type"=0.0, "Left RPM"=0.0, "Override RPM"=0, "Override Angle"=0, "Right RPM"=0.0, "Angle"=0.0, "Intake Mode"=0, "Intake Cmd"=0, "Intake O"=0, "Eject O"=0, "Angle O"=0, "Arm O"=0, "Intake Speed"=0.0, "Eject Speed"=0.0, "Arm Angle"=0.0, "Arm Speed"=0.0, "Intake?"=0, "Eject?"=0, "Left"=0.0, "Right"=0.0, "Pivot Speed"=0.0, "Y Dist"=0.0, "Position"=0.0, "Desired Position"=0, "Shooter Mode"=0.0, "Shooter Command"=0.0}, "Auton File Lists"={"Current Queue"="", "General Scripts"="", "Defense Scripts"="", "Movement Scripts"=""}, "Drivetrain Status Cluster"={"Modes"=enum."Manual", "Y (Throttle)"=0.0, "X (Steer)"=0.0, "Gyro In Range?"=FALSE, "Distance Drive Finished?"=FALSE, "Stop Eject Lockout"=FALSE, "Dist Drive Status"={"Y In Range"=FALSE, "X In Range"=FALSE, "Gyro In Range"=FALSE, "Y Dist"=0.0, "X Dist"=0.0, "Gyro"=0.0}, "Y Target"=0.0, "Heading Target"=0.0, "Vision Target Aligned?"=FALSE, "Gear"=0.0, "1st Gear Time"=0.0, "2nd Gear Time"=0.0, "1st Gear Shifts"=0.0, "2nd Gear Shifts"=0.0}, "Encoder Values"={"Left Encoder"={"Distance"=0.0, "Speed"=0.0, "Ticks"=0.0}, "Right Encoder"={"Distance"=0.0, "Speed"=0.0, "Ticks"=0.0}}, "IMU Data"={"Pitch"=0.0, "Roll"=0.0, "Yaw"=0.0, "Data Valid?"=FALSE, "Temp"=0.0, "MOVING"=FALSE, "YAW_STABLE"=FALSE, "Accel X"=0.0, "Accel Y"=0.0, "Accel Z"=0.0, "Accel Magnitude"=0.0, "Pitch Rate"=0.0, "Roll Rate"=0.0, "Yaw Rate"=0.0, "NavX Opened?"=FALSE, "Calibration Status"=0, "OP Status"=0}, "Power and Diagnostic Data"={"PDP Data"={"Battery Voltage"=0.0, "Temperature (degrees C)"=0.0, "Internal Battery R (Ohms)"=0.0, "Energy (J)"=0.0, "Power (W)"=0.0, "Total Current (A)"=0.0, "Battery Voltage Fault"=FALSE, "Temperature Fault"=FALSE, "Hardware Fault"=FALSE, "Currents"={"[0]"=0.0, "[1]"=0.0, "[2]"=0.0, "[3]"=0.0, "[4]"=0.0, "[5]"=0.0, "[6]"=0.0, "[7]"=0.0, "[8]"=0.0, "[9]"=0.0, "[10]"=0.0, "[11]"=0.0, "[12]"=0.0, "[13]"=0.0, "[14]"=0.0, "[15]"=0.0}, "Current Faults"={"[0]"=FALSE, "[1]"=FALSE, "[2]"=FALSE, "[3]"=FALSE, "[4]"=FALSE, "[5]"=FALSE, "[6]"=FALSE, "[7]"=FALSE, "[8]"=FALSE, "[9]"=FALSE, "[10]"=FALSE, "[11]"=FALSE, "[12]"=FALSE, "[13]"=FALSE, "[14]"=FALSE, "[15]"=FALSE}}, "PCM Data"={"Compressor Fault"=FALSE, "Solenoid Fault"=FALSE, "Compressor Enabled"=FALSE, "Hardware Fault"=FALSE, "Compressor Current"=0.0}, "roboRIO input voltage (V)"=0.0, "roboRIO input current (A)"=0.0, "3.3V Rail Short"=FALSE, "5 V Rail Short"=FALSE, "6 V Rail Short"=FALSE, "roboRIO Brownout"=FALSE, "Outputs Enabled?"=FALSE}, "Gyro"=0.0, "Shooter State Cluster"={"State"=enum."Idle", "Left RPM"=0.0, "Right RPM"=0.0, "Shooter Ready?"=FALSE, "Ball Loaded?"=FALSE, "Current Angle"=0.0, "Angle Motor Output"=0.0, "Trigger Output"=0.0, "Angle Ready?"=FALSE, "RPM Ready?"=FALSE, "Vision Ready?"=FALSE, "Ball Loaded?"=FALSE, "Mode"=enum."Manual", "Shot Type"=enum."Batter Shot", "Pot Height"=0.0, "Current Tripped Forward?"=FALSE, "Current Tripped Backward?"=FALSE, "Right Servo"=0, "Left Servo"=0, "IR Override"=FALSE, "Intake Danger?"=FALSE, "Intake Angle Ready?"=FALSE}, "Intake Status Cluster"={"Roller Power"=0.0, "Angle Power"=0.0, "Intake Mode"=enum."Auto", "Intake States"=enum."Idle", "Rollers Active?"=FALSE, "Current Height"=0.0, "Target Height"=0.0, "Encoder Raw Position"=0.0, "Forward Tripped?"=FALSE, "Backward Tripped?"=FALSE, "Override IR?"=FALSE}, "Ultrasonic Data"={"Left Ultrasonic"=0.0, "Right Ultrasonic"=0.0}, "Climb Status Cluster"={"Pull Power"=0.0, "Unpin Power"=0.0, "PTO Engaged?"=FALSE, "Climb Mode"=enum."Auto"}, "Loop Times"={"DT Loop Timer"=0, "Shooter Loop Timer"=0, "Intake Loop Timer"=0, "US Loop Timer"=0, "Auton File Loop Timer"=0}, "Pressure"=0.0, "Pressure Voltage"=0.0, "Auton Line Number"=0, "Autoshift Enabled"=FALSE}, binary string=w201) -> (value=w186:T54)  [unwired: 3 in, 2 out]
        n72 = Unbundle By Name(w204) -> ("Robot IP"=→"Robot IP":string, "Camera Addr"=→"Camera IP":string)
        n73 = Unbundle By Name(w186) -> ("Auton Command Cluster"=→"Auton Command Cluster":T7, "Auton File Lists"=→"Auton File Lists":T8, "Shooter State Cluster"=w177:T20, "Encoder Values"=→"Encoder Values":T12, "Drivetrain Status Cluster"=w146:T15, "IMU Data"=w171:T32, "Power and Diagnostic Data"=→"Power and Diagnostic Data":T41, "Gyro"=→"Gyro" →"Gyro 2":dbl, "Intake Status Cluster"=w185:T26, "Climb Status Cluster"=w179:T30, "Loop Times"=→"Loop Times":T48, "Ultrasonic Data"=→"Ultrasonic Data":T34, "Pressure"=→"Pressure":dbl, "Pressure Voltage"=→"Pressure Sensor Voltage":dbl, "Auton Line Number"=→"Line Number":i32, "Autoshift Enabled"=→"Auto Shift Enabled?":bool)
        "IMU Data" <- w171
        "Intake Status Cluster" <- w185
        "Climb Status Cluster" <- w179
        "Shooter State Cluster" <- w177
        "Drivetrain Status Cluster" <- w146
        n74 = Unbundle By Name(w177) -> ("Right RPM"=→"Right RPM":dbl, "Left RPM"=→"Left RPM":dbl, "Angle Ready?"=→"Angle Ready?":bool, "RPM Ready?"=→"RPM Ready?":bool, "Vision Ready?"=→"Vision Ready?":bool, "Ball Loaded?"=→"Ball Loaded?":bool, "Shooter Ready?"=→"Shooter Ready?":bool, "State"=w196:T21, "Mode"=w195:T22)
        n75 = Unbundle By Name(w146) -> ("Modes"=w162:T16, "Gear"=→"Gear":dbl)
        n76 = Unbundle By Name(w171) -> ("Calibration Status"=→"navX Calibration Status":T5)
        n77 = Unbundle By Name(w185) -> ("Intake States"=w166:T28, "Intake Mode"=w182:T27)
        n78 = case shown="\"Goal Vision Targeting\"" w162 {
          tunnel: ["Manual" "Climb" "Goal Target" "PID Drive" "Hybrid Drive"] -> w160
          tunnel: [u32 16711680 u32 16770560 u32 6618880 u32 9263615 u32 16743698] -> w161
          frame "Manual", Default {
          }
          frame "Climb" {
          }
          frame "Goal Vision Targeting" {
          }
          frame "PID Distance Drive" {
          }
          frame "Hybrid" {
          }
        }
        n79 = Unbundle By Name(w179) -> ("Climb Mode"=w153:T31)
        n80 = case shown="\"Shooter Ready\"" w196 {
          tunnel: ["Idle" "Warmup" "Shooter Ready" "Shooting"] -> w191
          tunnel: [u32 3381759 u32 16746240 u32 16711680 u32 6618880] -> w194
          frame "Idle", Default {
          }
          frame "Warmup" {
          }
          frame "Shooter Ready" {
          }
          frame "Shoot" {
          }
        }
        n81 = case shown="\"Go Hard or Go Home\"" w166 {
          tunnel: ["Idle" "Rolling Rollers" "Moving to Angle" "Escape Death"] -> w170
          tunnel: [u32 3381759 u32 16746240 u32 16711680 u32 14309887] -> w169
          frame "Idle", Default {
          }
          frame "Set roller speed" {
          }
          frame "Move to angle" {
          }
          frame "Go Hard or Go Home" {
          }
        }
        n82 = case shown="\"Auto\"" w195 {
          tunnel: ["Manual" "Safe" "Auto"] -> w199
          tunnel: [u32 16711680 u32 16770560 u32 6618880] -> w200
          frame "Manual", Default {
          }
          frame "Safe" {
          }
          frame "Auto" {
          }
        }
        n83 = case shown="\"Semi-Auto\"" w153 {
          tunnel: ["Manual" "Auto" "Semi-Auto"] -> w157
          tunnel: [u32 16711680 u32 6618880 u32 16770560] -> w154
          frame "Manual", Default {
          }
          frame "Auto" {
          }
          frame "Semi-Auto" {
          }
        }
        n84 = case shown="\"Safe\"" w182 {
          tunnel: ["Manual" "Safe" "Auto"] -> w180
          tunnel: [u32 16711680 u32 16770560 u32 6618880] -> w183
          frame "Manual", Default {
          }
          frame "Safe" {
          }
          frame "Auto" {
          }
        }
        n85 = Bundle(w161, w161) -> (w158:cluster{u32, u32})  [unwired: 1 in]
        n86 = Build Array(w158) -> (w159:cluster{u32, u32}[])
        n87 = Bundle(w200, w200) -> (w197:cluster{u32, u32})  [unwired: 1 in]
        n88 = Bundle(w169, w169) -> (w168:cluster{u32, u32})  [unwired: 1 in]
        n89 = Bundle(w194, w194) -> (w193:cluster{u32, u32})  [unwired: 1 in]
        n90 = Build Array(w168) -> (w167:cluster{u32, u32}[])
        n91 = Build Array(w197) -> (w198:cluster{u32, u32}[])
        n92 = Bundle(w154, w154) -> (w155:cluster{u32, u32})  [unwired: 1 in]
        n93 = Build Array(w193) -> (w192:cluster{u32, u32}[])
        n94 = property on="Drivetrain Mode" class="Bool (strict)"("BoolText.Text"=w160, "Colors [4]"=w159) -> ()  [unwired: 2 in, 2 out]
        n95 = property on="Intake State" class="Bool (strict)"("Colors [4]"=w167, "BoolText.Text"=w170) -> ()  [unwired: 2 in, 2 out]
        n96 = Bundle(w183, w183) -> (w184:cluster{u32, u32})  [unwired: 1 in]
        n97 = property on="Shooter Mode" class="Bool (strict)"("BoolText.Text"=w199, "Colors [4]"=w198) -> ()  [unwired: 2 in, 2 out]
        n98 = Build Array(w155) -> (w156:cluster{u32, u32}[])
        n99 = property on="Shooter State" class="Bool (strict)"("BoolText.Text"=w191, "Colors [4]"=w192) -> ()  [unwired: 2 in, 2 out]
        n100 = Build Array(w184) -> (w181:cluster{u32, u32}[])
        n101 = property on="Climb Mode" class="Bool (strict)"("BoolText.Text"=w157, "Colors [4]"=w156) -> ()  [unwired: 2 in, 2 out]
        n102 = property on="Intake Mode" class="Bool (strict)"("BoolText.Text"=w180, "Colors [4]"=w181) -> ()  [unwired: 2 in, 2 out]
        "Control Info" <- w207
        "Status Info" <- w206
        "Robot Metrics" <- w205
        "DS TCP" <- w204
      }
    }
  }
  n103 = while {
    stop <- FALSE stop-if-true
    n104 = Bundle By Name(cluster=T55 {"Shooter Presets"={"Batter Shot"={"L"=0.0, "R"=0.0, "A"=0.0}, "Deep Middle"={"L"=0.0, "R"=0.0, "A"=0.0}, "Manual Shot"={"L"=0.0, "R"=0.0, "A"=0.0}, "Left Ticks Per Rotation"=0.0, "Right Ticks Per Rotation"=0.0, "Low Bar Shot"={"L"=0.0, "R"=0.0, "A"=0.0}, "Shooter RPM Tolerance"=0.0, "Trigger Power"=0.0, "Fire from Load Delay"=0, "Max Angle"=0.0, "Min Angle"=0.0, "Angle PID gains"={"P"=1.0, "I"=0.01, "D"=0.0}, "Angle Output"={"output high"=0.0, "output low"=0.0}, "Shooter Angle Tolerance"=0.0, "Vision Shoot x^2"=0.0, "Vision Shoot x"=0.0, "Feed Forward Max Accel"=0.0, "Feed Forward Kv"=0.0, "Backwards Trigger"=0.0, "Shot Finish Delay (ms)"=0.0, "Angle Max Current"=0.0, "Angle Current Trip Time"=0.0, "Intake Angle"=0.0, "Vision Shoot c"=0.0, "Reset?"=FALSE, "Button Release Delay"=0.0, "Angle Pot x"=0.0, "Angle Pot c"=0.0, "Ignore Angle?"=FALSE, "Max RPM"=0.0, "Safty Frist Angle"=0.0, "Intake Danger Height"=0.0, "Angle Pot B"=0, "Angle Pot M"=0.0, "FF Finish RPM"=0.0, "RPM PID Right"={"P"=1.0, "I"=0.01, "D"=0.0, "FF"=0.0}, "RPM PID Left"={"P"=1.0, "I"=0.01, "D"=0.0, "FF"=0.0}, "Backwards RPM"=0.0, "Vision RPM"=0.0, "Run Wheels Backward Delay"=0, "Cleat Shot"={"L"=0.0, "R"=0.0, "A"=0.0}, "Vision Far RPM"=0.0, "Vision Far Distance"=0.0, "Vision Far Angle"=0.0}, "Encoder Control"={"Right Tick Constant"=0.0, "Left Tick Constant"=0.0, "Reset?"=FALSE, "Y Dist"={"PID gains"={"proportional gain (Kc)"=0.0, "integral time (Ti, min)"=0.0, "derivative time (Td, min)"=0.0}}, "Y Stop Thresh"=0.0, "Y Stop Speed"=0.0}, "Steer PID output"={"output high"=0.0, "output low"=0.0}, " Steer PID gains"={"proportional gain (Kc)"=0.0, "integral time (Ti, min)"=0.0, "derivative time (Td, min)"=0.0}, "Drivetrain Settings"={"Gyro Tolerance"=0.0, "Throttle Ramp (ms)"=0.0, "Kv"=0.0, "Ka"=0.0, "Feed Forward P"=0.0, "Feed Forward D"=0.0, "Goal Vision PID gains"={"proportional gain (Kc)"=1.0, "integral time (Ti, min)"=0.01, "derivative time (Td, min)"=0.0}, "Goal Detection Window"=0.0, "Creep Rate"=0.0, "Vision Throttle Threshold"=0.0, "Min Turn Output"=0.0, "Left Batter Angle"=0.0, "Right Batter Angle"=0.0}, "Vision Packet"={"Distance"=0.0, "Center X"=0.0, "Center Y"=0.0, "Found Target?"=FALSE, "Robot Center"=0.0, "Angle"=0.0}, "Dashboard Drivetrain Command"={"Drivetrain Vision"={"Goal Window"=0.0, "Ball Window"=0.0}}, "Info/Command Cluster"={"Distance to Ball"=0.0, "Desired Angle"=0.0, "Command"=enum."Turn to Ball", "Pixels from Center"=0.0}, "Ball Vision Packet"={"Ball Detected?"=FALSE, "Distance to Ball"=0.0, "Desired Angle"=0.0, "Pixels from Center"=0.0, "Tracking mode"=enum."Turn to Ball"}, "Intake Presets"={"Intake Speed"=0.0, "Outake Speed"=0.0, "Low Height"=0.0, "Half Height"=0.0, "High Idle Height"=0.0, "Angle Speed"=0.0, "Angle Tolerance"=0.0, "Encoder Scale"=0.0, "Load Height"=0.0, "Output Range"={"output high"=0.0, "output low"=0.0}, "Rotation Power Max/Min"=0.0, "MaxCurrent"=0.0, "Intake Trip Time"=0.0, "Idle Height"=0.0, "Max Height"=0.0, "Reset Encoders?"=FALSE, "PID gains"={"proportional gain (Kc)"=0.0, "integral time (Ti, min)"=0.0, "derivative time (Td, min)"=0.0}, "Intake Stop Delay"=0, "Settle Time"=0.0, "Settle Wait Time"=0.0, "Pull Up Delay"=0.0}, "Intake Encoder Control"={"Arm Tick Constant"=0.0, "Reset?"=FALSE, "Y Dist"={"PID gains"={"proportional gain (Kc)"=0.0, "integral time (Ti, min)"=0.0, "derivative time (Td, min)"=0.0}}, "Y Stop Thresh"=0.0, "Y Stop Speed"=0.0}, "Climb Presets"={"Pull Power"=0.0, "Extend Power"=0.0}, "Goal Output Range"={"output high"=0.0, "output low"=0.0}, "Enabled Systems"={"Shoot"=TRUE, "Intake"=TRUE, "DT"=TRUE, "Gyro"=TRUE, "100ms"=TRUE, "US"=TRUE}, "Auton Presets"={"Pitch Limit"=0.0, "Roll Limit"=0.0, "Start Position"=0.0, "Cross Position"=0.0}, "Pressure M"=0.0, "Pressure B"=0.0, "Vision Timeout"=0.0, "Auto-Shift"={"Delay"=0.0, "Speed Thresh"=0.0, "Upshift Accel"=0.0, "Upshift Throttle"=0.0, "Upshift Throttle Accel"=0.0, "Downshift Throttle"=0.0, "Downshift Throttle Accel"=0.0}} ("anything"), "Auto-Shift"="Auto-Shift", "Shooter Presets"="Shooter Presets", "Goal Output Range"="Goal Output Range", "Drivetrain Settings"="Drivetrain Settings", "Steer PID output"="Steer PID output", "Steer PID gains"="Steer PID gains", "Intake Presets"="Intake Presets", "Climb Presets"="Climb Presets", "Encoder Control"="Encoder Settings", "Auton Presets"="Auton Presets", "Pressure M"="Pressure M", "Pressure B"="Pressure B", "Vision Timeout"="Vision Timeout") -> (w266:T55)
    n105 = Flatten To String(anything=w266) -> (data string=w268:string)  [unwired: 3 in, 2 out]
    n106 = Wait (ms)(milliseconds to wait=u32 250) -> ()  [unwired: 1 out]
    n107 = local read "Robot IP"() -> (w270:string)
    n108 = call "DumbDash Send.vi"("Robot IP"=w270, "data string"=w268) -> ()  [unwired: 10 in]
  }
  n109 = while {
    tunnel: w29 -> [w279]
    shift-right: [w271] -> _
    shift-left: w28 -> [w278]
    tunnel: [w277] -> _
    tunnel: w24 -> [w276]
    tunnel: w23 -> [w275]
    tunnel: w22 -> [_]
    tunnel: w19 -> [w274]
    shift-right: [w272] -> _
    shift-left: _ -> [w273]
    i -> [w277]
    stop <- FALSE stop-if-true
    n110 = event shown="[0] \"Rec Mode\": Value Change" {
      selector: w275 -> [_ _ _]
      dyn-events: [w283 _ _] -> _
      timeout: _ -> [_ _ _]
      tunnel: w279 -> [_ _ _]
      tunnel: w278 -> [w288 _ _]
      tunnel: w276 -> [w287 _ w301]
      tunnel: w274 -> [w286 _ _]
      tunnel: w273 -> [_ _ _]
      tunnel: [0 _ _] -> w272
      tunnel: [w288 _ _] -> w271
      event "Rec Mode": Value Change {
        n111 = event-data() -> ("NewVal"=w281:enum32{"Stop", "Record", "Playback"})  [unwired: 1 in]
        n112 = case shown="\"Playback\"" w281 {
          tunnel: w287 -> [_ w291 w295]
          tunnel: [_ _ w299] -> w283
          tunnel: [_ _ w298] -> _
          tunnel: w286 -> [_ _ w293]
          tunnel: cluster{i32, i32} {-250, 170} -> [_ _ w292]
          tunnel: [_ _ T63 {"Image Size"=TRUE, "Image Type"=TRUE, "Pixel Value"=TRUE, "ROI Information"=TRUE, "Zoom Factor"=FALSE} ("Image Information Shown:All Elements")] -> _
          tunnel: [_ _ TRUE ("Zoom Factor")] -> _
          frame Default {
          }
          frame "Stop", "Record" {
            # "Place Window too"
            n113 = invoke class="VI" method="FP.Close"(reference=w291) -> (reference out=w290:refnum<vi>)  [unwired: 2 in, 2 out]
            n114 = invoke class="VI" method="Abort VI"(reference=w290) -> ()  [unwired: 2 in, 3 out]
          }
          frame "Playback" {
            n115 = call "Open Playback Panel.vi"("Offset"=w292, "DB VI Ref"=w293, "Playback in"=w295) -> ("Playback out"=w294:refnum<vi>)  [unwired: 8 in]
            n116 = register-events(w294) -> (reference out=w299:refnum<event-registration>, error out=w298:errorcluster)  [unwired: 2 in]
          }
        }
        n117 = global write "WPI_DashboardLogging Global.vi" "Logging Filename"(path "") -> ()
        n118 = global write "WPI_DashboardLogging Global.vi" "Recording"(w281) -> ()
        n119 = call <vilib>:"WPI_DashboardNT Log FieldName Cache.vi"("Operation"=enum16{"Lookup/Add", "Index", "Clear"}."Clear") -> ()  [unwired: 8 in, 3 out]
      }
      event Panel Close {
        w300 = enum32{"Stop", "Record", "Playback"}."Stop" ("Rec Mode")
        n120 = event-data() -> ()  [unwired: 1 in, 4 out]
        n121 = local write "Rec Mode"(w300) -> ()
        n122 = global write "WPI_DashboardLogging Global.vi" "Recording"(w300) -> ()
      }
      event Panel Close {
        n123 = event-data() -> ()  [unwired: 1 in, 4 out]
        n124 = invoke class="VI" method="FP.Close"(reference=w301) -> (reference out=w303:refnum<vi>)  [unwired: 2 in, 2 out]
        n125 = invoke class="VI" method="Abort VI"(reference=w303) -> (error out=w302:errorcluster)  [unwired: 2 in, 2 out]
        n126 = invoke class="VI" method="Abort VI"(error in=w302) -> ()  [unwired: 2 in, 3 out]
      }
    }
  }
  n127 = property class="Pnl"(reference=w26) -> ("Panes[]"=w27:refnum<vi>[])  [unwired: 1 in, 2 out]
  n128 = Index Array(array=w27) -> (element=w25:refnum<vi>)  [unwired: 1 in]
  n129 = while {
    tunnel: w25 -> [w305]
    i -> [w308]
    stop <- FALSE stop-if-true
    n130 = Wait (ms)(milliseconds to wait=u32 100) -> ()  [unwired: 1 out]
    n131 = case shown="\"Record\"" "Rec Mode" {
      tunnel: w308 -> [_ _ w323]
      tunnel: [u32 2829099 ("Base Color") u32 11141120 ("Target Color") w312] -> w304
      frame "Stop", Default {
        # "Reset the color, extra updates don't cost much"
      }
      frame "Record" {
      }
      frame "Playback" {
        # "Playback"
        n132 = Quotient & Remainder(x=w323, y=u32 50 ("milliseconds to wait")) -> (x-y*floor(x/y)=w319:u32)  [unwired: 1 out]
        n133 = Divide(x=w319, y=u32 50 ("milliseconds to wait")) -> (x/y=w316:dbl)
        n134 = Multiply(x=6.283185307179586, y=w316) -> (x*y=w321:dbl)
        n135 = Sine(x=w321) -> (sin(x)=w320:dbl)
        n136 = Absolute Value(x=w320) -> (abs(x)=w313:dbl)
        n137 = call "Interpolate RGB Color.vi"("Proportion"=w313, "Target Color"=u32 30976, "Base Color"=u32 2829099) -> ("Result Color"=w312:u32)  [unwired: 8 in]
      }
    }
    n138 = property class="Pane"(reference=w305, "PaneColor"=w304) -> ()  [unwired: 1 in, 2 out]
  }
  n139 = global write "WPI_DashboardLogging Global.vi" "Recording"(w10) -> ()
  n140 = local write "Rec Mode"(w10) -> ()
  n141 = disable-structure shown="Disabled" {
    frame Disabled {
      w326 = T49 4 items=["Grayscale (U8)", "Grayscale (I16)", "Grayscale (SGL)", "Complex (CSG)", "RGB (U32)", "HSL (U32)", "RGB (U64)", "Grayscale (U16)"] ("Image Type")
      n142 = call "IMAQ Create"("Image Name"="Ball Watcher", "Image Type"=w326) -> ("New Image"=w324:T4)  [unwired: 3 in, 1 out]
      n143 = while {
        tunnel: w324 -> [w328]
        stop <- FALSE stop-if-true
        n144 = local read "Camera IP"() -> (w334:string)
        n145 = local read "Rec Mode"() -> (w335:enum32{"Stop", "Record", "Playback"})
        n146 = call "624WPI_CameraRead MJPG for Dashboard.vi"("Camera Settings"="Ball Camera Settings", "Rec Mode"=w335, "Camera IP"=w334, "Camera Mode"="Camera Mode 2", "Refnum in"=w328) -> ("Active"=w336:bool, "Refnum out"=w330:T4, "FPS"=w331:dbl, "Bandwidth (Mbps)"=w332:dbl)  [unwired: 3 in]
        "Ball Cam Active?" <- w336
        n147 = case shown="True" w336 {
          tunnel: w330 -> [_ w338]
          tunnel: w331 -> [_ w340]
          tunnel: w332 -> [_ w339]
          frame False {
            n148 = Wait Until Next ms Multiple(millisecond multiple=u32 500) -> ()  [unwired: 1 out]
          }
          frame True {
            "Front Camera Display 2" <- w338
            "FPS 2" <- w340
            "Bandwidth (Mbps) 2" <- w339
            "Front Camera Display 3" <- w338
          }
        }
      }
    }
    frame Enabled {
    }
  }
  n149 = while {
    tunnel: u16 1741 ("timeout ms (25000)") -> [w342]
    stop <- FALSE stop-if-true
    n150 = TCP Create Listener(10:w342) -> (0:w341:errorcluster, 3:w343:refnum<k5>)  [unwired: 4 in, 1 out]
    n151 = case shown="No Error" w341 {
      selector: w341 -> [w345 _]
      tunnel: w343 -> [w346 _]
      frame No Error {
        n152 = while {
          tunnel: w346 -> [w349]
          tunnel: w345 -> [w348]
          stop <- FALSE stop-if-true
          n153 = TCP Wait On Listener(8:w348, 11:w349) -> (0:w350:errorcluster, 4:w351:refnum<k5>)  [unwired: 2 in, 3 out]
          n154 = local write "TCP"(w351) -> ()
          n155 = case shown="No Error" w350 {
            frame No Error {
            }
            frame Error {
              n156 = Wait (ms)(milliseconds to wait=u32 1000) -> ()  [unwired: 1 out]
            }
          }
        }
      }
      frame Error {
        n157 = Wait (ms)(milliseconds to wait=u32 1000) -> ()  [unwired: 1 out]
      }
    }
  }
  n158 = call <vilib>:"Intialize Keyboard.vi"() -> ("device ID"=w9:refnum<k1>)  [unwired: 10 in, 1 out]
  n159 = while {
    stop <- FALSE stop-if-true
    n160 = local read "IMU Data"() -> (w365:T32)
    n161 = local read "Mode"() -> (w361:T3)
    n162 = Unbundle By Name(w365) -> ("Data Valid?"=w364:bool)
    n163 = Equal?(x=w361, y=T3."Disconnected") -> (x = y?=w358:bool)
    n164 = Equal?(x=w361, y=T3."No Code") -> (x = y?=w359:bool)
    n165 = Or(x=w358, y=w359) -> (x .or. y?=w360:bool)
    n166 = Or(x=w364, y=w360) -> (x .or. y?=w357:bool)
    n167 = case shown="False" w357 {
      tunnel: [w366 u32 2829099 ("Base Color")] -> w354
      frame False {
        n168 = Tick Count (ms)() -> (millisecond timer value=w367:u32)
        n169 = Quotient & Remainder(x=w367, y=u32 1000 ("milliseconds to wait")) -> (x-y*floor(x/y)=w374:u32)  [unwired: 1 out]
        n170 = Divide(x=w374, y=u32 1000 ("milliseconds to wait")) -> (x/y=w371:dbl)
        n171 = Multiply(x=6.283185307179586, y=w371) -> (x*y=w376:dbl)
        n172 = Sine(x=w376) -> (sin(x)=w375:dbl)
        n173 = Absolute Value(x=w375) -> (abs(x)=w370:dbl)
        n174 = call "Interpolate RGB Color.vi"("Proportion"=w370, "Target Color"=u32 16711680, "Base Color"=u32 2829099) -> ("Result Color"=w366:u32)  [unwired: 8 in]
      }
      frame True {
      }
    }
    n175 = property on="Gyro" class="Knob (strict)"("BGColor"=w354) -> ()  [unwired: 2 in, 2 out]
    n176 = property on="Gyro 2" class="Knob (strict)"("BGColor"=w354) -> ()  [unwired: 2 in, 2 out]
    n177 = Wait (ms)(milliseconds to wait=u32 50) -> ()  [unwired: 1 out]
  }
  n178 = while {
    tunnel: w9 -> [w383]
    stop <- FALSE stop-if-true
    n179 = local read "Robot IP"() -> (w381:string)
    n180 = call-poly <vilib>:"Acquire Input Data.vi"("device ID"=w383) -> ("keys pressed"=w382:T64)  [unwired: 16 in, 2 out]
    n181 = call "Send Keyboard Data.vi"("Robot IP"=w381, "keys pressed"=w382) -> ()  [unwired: 10 in]
    n182 = Wait (ms)(milliseconds to wait=50) -> ()  [unwired: 1 out]
  }
  n183 = global write "WPI_DashboardLogging Global.vi" "Recording"(w20) -> ()
  n184 = local write "Rec Mode"(w20) -> ()
  n185 = control-ref of="Dashboard Tab"() -> (w1:refnum<vi>)
  n186 = call "DumbDash Load Controls.vi"("TabControl in"=w1) -> ("Array"=w12:T65[])  [unwired: 10 in]
  n187 = control-ref of="DumbDashMessage"() -> (w11:refnum<vi>)
  n188 = while {
    tunnel: w12 -> [w389]
    tunnel: w11 -> [w387]
    stop <- FALSE stop-if-true
    n189 = disable-structure shown="Enabled" {
      disable-tunnel: ["Robot" Robot_Name."Main Robot" ("Robot")] -> w384
      frame Disabled {
      }
      frame Enabled {
      }
    }
    n190 = Wait (ms)(milliseconds to wait=u32 250) -> ()  [unwired: 1 out]
    n191 = disable-structure shown="RUN_TIME_ENGINE==True" {
      disable-tunnel: "stop" -> [w394 w395]
      frame condition #0 {
        # "Close the build DB"
        n192 = Quit LabVIEW(quit? (T)=w394) -> ()
      }
      frame condition #1 (active) {
        n193 = Stop(stop? (T)=w395) -> ()
      }
    }
    n194 = case shown="True" "Save" {
      tunnel: w389 -> [_ w405]
      tunnel: w387 -> [_ w404]
      tunnel: w384 -> [_ w403]
      frame False {
      }
      frame True {
        n195 = flat-sequence {
          tunnel: w405 -> [w408]
          tunnel: w404 -> [w407]
          tunnel: w403 -> [w406]
          frame #0 {
            n196 = call "DumbDash Save Values.vi"("Message Box"=w407, "Robot"=w406, "Controls In"=w408) -> ()  [unwired: 9 in]
          }
          frame #1 {
            n197 = local write "Save"(FALSE) -> ()
          }
        }
      }
    }
    n198 = case shown="True" "Load" {
      tunnel: w389 -> [_ w398]
      tunnel: w387 -> [_ w397]
      tunnel: w384 -> [_ w396]
      frame False {
      }
      frame True {
        n199 = flat-sequence {
          tunnel: w398 -> [w401]
          tunnel: w397 -> [w400]
          tunnel: w396 -> [w399]
          frame #0 {
            n200 = call "DumbDash Load Values.vi"("Message Box"=w400, "Robot"=w399, "Controls In"=w401) -> ()  [unwired: 9 in]
          }
          frame #1 {
            n201 = local write "Load"(FALSE) -> ()
          }
        }
      }
    }
  }
  n202 = local write "Load"(TRUE) -> ()
